vi "SQL_Test_Data_SelectByTime.vi"(7 "结束时间":timestamp=timestamp(3516339005.4444437 s since 1904-01-01), 8 "起始时间":timestamp=timestamp(3515993400.420156 s since 1904-01-01), 9 "通道名":string="声发射") -> (0 "x-y":u32, 1 "error out":errorcluster, 3 "数据":dbl[](array[numeric]))   [LabVIEW 2014]
uses:
  <vilib>/addons/database/Connection.llb/DB Tools Open Connec (String).vi
  <vilib>/addons/database/_DB Variant To Data/Database Variant To Data.xnode
  <vilib>/addons/database/NI_Database_API.lvlib
panel:
  out "数据":dbl[](array[numeric])
  out "时间":timestamp[](array[timestamp])
  out "行数":i32
  in  "类型数组":cluster{timestamp, string}[](array[cluster])
  out "毫秒计时值":u32
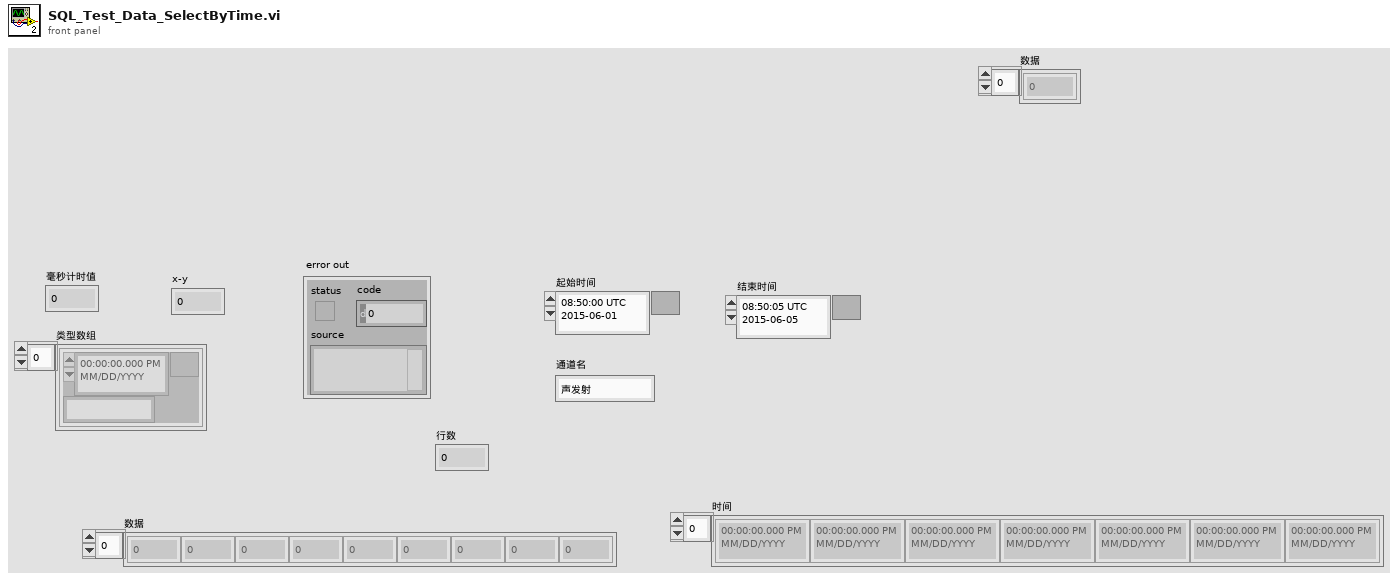
[diagram p1: front panel]
types:
  T1 = typedef "NI_Database_API.lvlib/Conn ObjectReference.ctl" = refnum<k1>
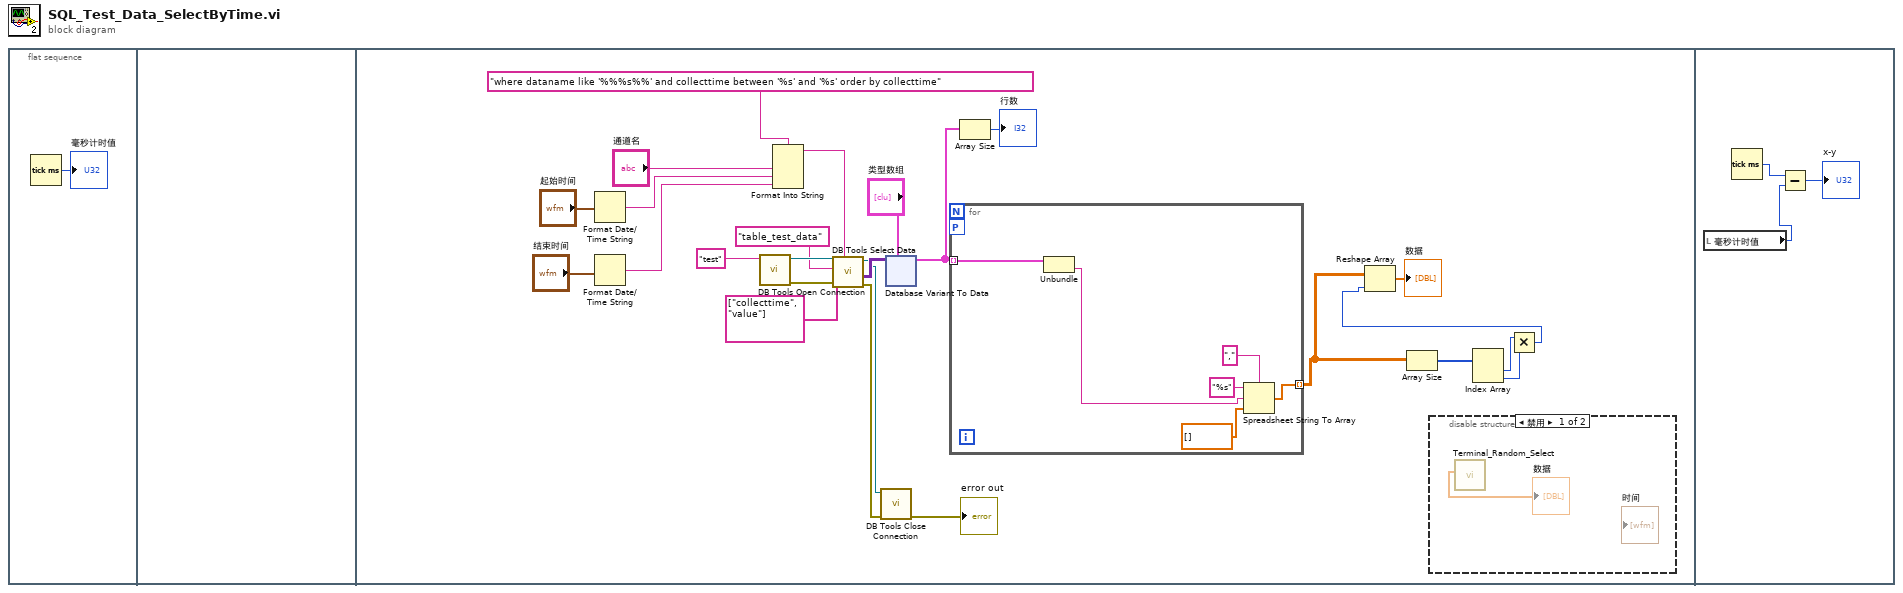
[diagram p0: block diagram]
diagram:
  n1 = flat-sequence {
    frame #0 {
      n2 = Tick Count (ms)() -> (millisecond timer value=→"毫秒计时值":u32)
    }
    frame #1 {
    }
    frame #2 {
      n3 = Format Date/Time String(seconds (now)="起始时间") -> (date/time string=w13:string)  [unwired: 2 in]
      n4 = Format Date/Time String(seconds (now)="结束时间") -> (date/time string=w11:string)  [unwired: 2 in]
      n5 = call-poly <vilib>:"DB Tools Open Connection.vi"("connection information"="test") -> ("error out"=w24:errorcluster, "connection reference"=w25:T1)  [unwired: 7 in]
      n6 = Format Into String(format string="where dataname like '%%%s%%' and collecttime between '%s' and '%s' order by collecttime" ("condition"), "通道名", w13, w11) -> (resulting string=w10:string)  [unwired: 2 in, 1 out]
      n7 = call <vilib>:"DB Tools Select Data.vi"("condition"=w10, "error in (no error)"=w24, "columns"=string[] ["collecttime", "value"], "table"="table_test_data", "connection reference"=w25) -> ("error out"=w19:errorcluster, "data"=w22:variant[][], "connection reference out"=w20:T1)  [unwired: 1 in]
      n8 = call <vilib>:"DB Tools Close Connection.vi"("error in (no error)"=w19, "connection reference"=w20) -> ("error out"=→"error out":errorcluster)  [unwired: 5 in]
      n9 = xnode "Database Variant To Data"("database variant"=w22, "type"="类型数组") -> ("data"=w9:cluster{timestamp, string}[])  [unwired: 1 in, 1 out]
      n10 = for "For循环" {
        tunnel: w9 -> [w30] mode=indexing
        tunnel: [w29] -> w7 mode=indexing
        workers-P: _ -> [_]
        n11 = Unbundle(w30) -> (w28:string)  [unwired: 1 out]
        n12 = Spreadsheet String To Array(delimiter (Tab)="," ("分隔符(Tab)"), format string="%s" ("格式字符串"), spreadsheet string=w28, array type (2D Dbl)=dbl[] [] ("数组类型(2D Dbl)")) -> (array=w29:dbl[])
      }
      n13 = Array Size(array=w9) -> (size(s)=→"行数":i32)
      n14 = Array Size(array=w7) -> (size(s)=w6:i32[])
      n15 = disable-structure shown="禁用" {
        frame Disabled {
          n16 = call "Terminal_Random_Select.vi"() -> ("添加的数组"=→"数据":dbl[])  [unwired: 10 in]
        }
        frame Enabled {
        }
      }
      n17 = Index Array(array=w6) -> (element #1=w5:i32, element #2=w4:i32)  [unwired: 2 in]
      n18 = Multiply(x=w5, y=w4) -> (x*y=w3:i32)
      n19 = Reshape Array(w7, w3) -> (→"数据":dbl[])
    }
    frame #3 {
      n20 = local read "毫秒计时值"() -> (w120:u32)
      n21 = Tick Count (ms)() -> (millisecond timer value=w121:u32)
      n22 = Subtract(x=w121, y=w120) -> (x-y=→"x-y":u32)
    }
  }
